vi "HTTP Post.vi"(4 "Password":string="border", 6 "UserName":string="admin", 7 "Host":string="192.168.1.202:2002/jpg/image.jpg", 8 "error in (no error)":errorcluster, 10 "Body In":string, 11 "Header In":T1[](array[typedef])) -> (0 "error out":errorcluster, 2 "Body Out":string, 3 "Header Out":T1[](array[typedef]))   [LabVIEW 2014]
uses:
  Documents/sw-lv/@Menu/Controlli/Command Structure.ctl
  <vilib>/httpClient/POSTBuffer.vi
  <vilib>/httpClient/LabVIEWHTTPClient.lvlib
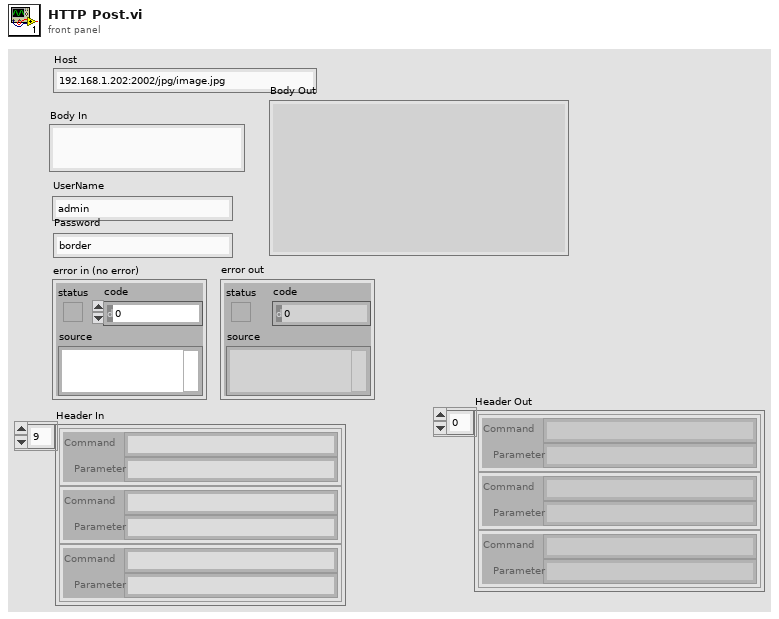
[diagram p1: front panel]
types:
  T1 = typedef "Command Structure.ctl" = cluster{"Command":string, "Parameter":string}
  T2 = typedef "LabVIEWHTTPClient.lvlib/ClientHandle.ctl" = refnum<k1>
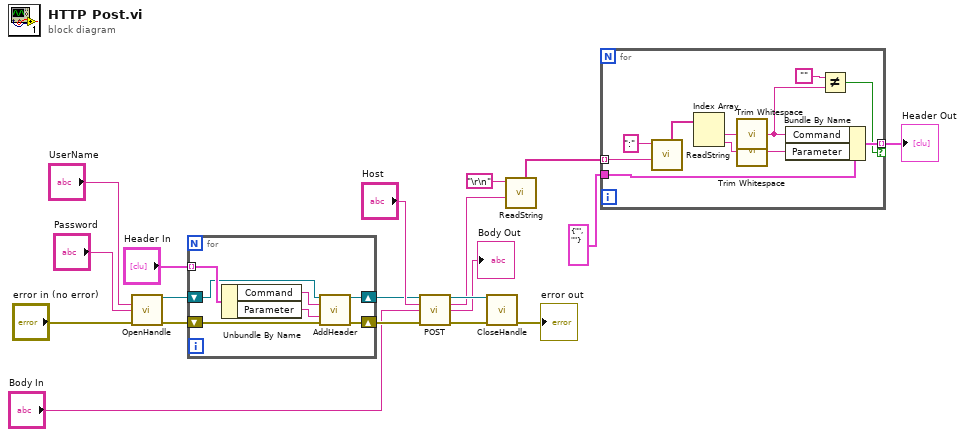
[diagram p0: block diagram]
diagram:
  n1 = call <vilib>:"OpenHandle.vi"("username"="UserName", "password"="Password", "error in (no error)"="error in (no error)") -> ("client handle out"=w5:T2, "error out"=w4:errorcluster)  [unwired: 11 in]
  n2 = for {
    tunnel: "Header In" -> [w26] mode=indexing
    shift-right: [w20] -> w3
    shift-left: w5 -> [w23]
    shift-right: [w22] -> w2
    shift-left: w4 -> [w21]
    n3 = Unbundle By Name(w26) -> ("Command"=w25:string, "Parameter"=w24:string)
    n4 = call <vilib>:"AddHeader.vi"("client handle"=w23, "header"=w25, "value"=w24, "error in (no error)"=w21) -> ("client handle out"=w20:T2, "error out"=w22:errorcluster)  [unwired: 10 in]
  }
  n5 = call-poly <vilib>:"POST.vi"("client handle"=w3, "url"="Host", "buffer"="Body In", "error in (no error)"=w2) -> ("client handle out"=w17:T2, "headers"=w12:string, "body"=→"Body Out":string, "error out"=w16:errorcluster)  [unwired: 8 in]
  n6 = call <vilib>:"CloseHandle.vi"("client handle"=w17, "error in (no error)"=w16) -> ("error out"=→"error out":errorcluster)  [unwired: 13 in]
  n7 = call "ReadString.vi"("Separatore"="\r\n", "InString"=w12) -> ("String Array"=w10:string[])  [unwired: 3 in, 3 out]
  n8 = for {
    tunnel: w10 -> [w37] mode=indexing
    tunnel: T1 {"Command"="", "Parameter"=""} ("LV Command Structure") -> [w34]
    tunnel: [w32] -> w8 mode=indexing if=w28
    n9 = call "ReadString.vi"("Separatore"=":", "InString"=w37) -> ("String Array"=w35:string[])  [unwired: 3 in, 3 out]
    n10 = Index Array(array=w35) -> (element #1=w31:string, element #2=w33:string)  [unwired: 2 in]
    n11 = call <vilib>:"Trim Whitespace.vi"("string"=w31) -> ("trimmed string"=w30:string)  [unwired: 1 in]
    n12 = call <vilib>:"Trim Whitespace.vi"("string"=w33) -> ("trimmed string"=w27:string)  [unwired: 1 in]
    n13 = Bundle By Name(cluster=w34, "Command"=w30, "Parameter"=w27) -> (w32:T1)
    n14 = Not Equal?(x="", y=w30) -> (x != y?=w28:bool)
  }
  "Header Out" <- w8
